vi "Stop Core.vi"(10 "final error code":i32, 11 "CS++SeqEditor in":refnum<class "CS++SeqEditor.lvclass">) -> (3 "CS++SeqEditor out":refnum<class "CS++SeqEditor.lvclass">)   [LabVIEW 2016, in "CS++SeqEditor.lvlib" / "CS++SeqEditor.lvclass"]
doc: "(<B>Filename</B>: Actor Framework.lvlib:Actor.lvclass:Stop Core.vi)\n\nDefines what the actor does before it stops. Use the <B>final error code</B> input to determine whether the actor shut down in response to an error.\n\nBy default, this method does nothing. A descendant class may override it to define behavior, such as shutting down any processes the actor initiated in its override of the Actor Core method."
uses:
  CS++SeqEditor.lvclass
  CS++SeqEditor.lvclass/CS++SeqEditor.ctl
  CSPP_Core/Actors/CS++GUIActor/CS++GUIActor.lvclass
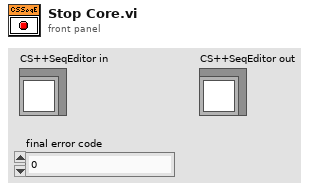
[diagram p1: front panel]
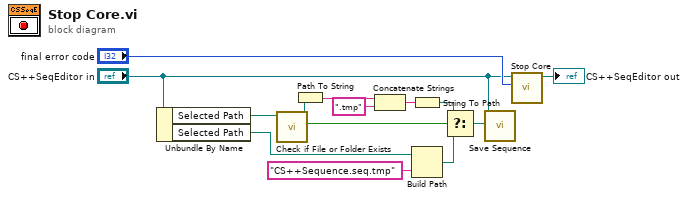
[diagram p0: block diagram]
diagram:
  n1 = Unbundle By Name("CS++SeqEditor in") -> ("Selected Path"=w12:path, "Selected Path"=w6:path)
  n2 = call <vilib>:"Check if File or Folder Exists.vi"("path"=w12) -> ("file or folder exists?"=w11:bool, "dup path"=w10:path)  [unwired: 8 in, 1 out]
  n3 = Path To String(path=w10) -> (string=w9:string)
  n4 = Concatenate Strings(w9, ".tmp" ("string")) -> (w7:string)
  n5 = String To Path(string=w7) -> (path=w4:path)
  n6 = Build Path(base path=w6, name or relative path="CS++Sequence.seq.tmp") -> (appended path=w3:path)
  n7 = Select(t=w4, s=w11, f=w3) -> (s? t:f=w2:path)
  n8 = call "Save Sequence.vi"("Selected Path"=w2, "CS++SeqEditor in"="CS++SeqEditor in") -> ()  [unwired: 8 in, 2 out]
  n9 = call-parent "Stop Core.vi"("final error code"="final error code", "CS++GUIActor in"="CS++SeqEditor in") -> ("CS++GUIActor out"=→"CS++SeqEditor out":refnum<class "CS++SeqEditor.lvclass">)  [unwired: 9 in]
